vi "Error - Fire Error.vi"(8 "error in (no error)":errorcluster, 10 "Error Type":T1, 11 "View Model":T2) -> (0 "error out":errorcluster, 3 "View Model":T2)   [LabVIEW 2013]
doc: "Used to send errors to the error handling process."
uses:
  View Model/Controls/View Model.ctl
  Controls/Error Model.ctl
  Controls/Error Types.ctl
  View Model/Controls/Shared Model.ctl
  Elevator Controller/Controls/Elevator Model.ctl
  Elevator Controller/Controls/Controller Overhead.ctl
  Elevator Controller/Controls/Elevator States.ctl
  Elevator Controller/Controls/Elevator Location.ctl
  Elevator Controller/Controls/Elevator Command Event.ctl
  Elevator Controller/Controls/Elevator Commands.ctl
  Configuration/Controls/Configuration Model.ctl
  Configuration/Controls/Configuration Data.ctl
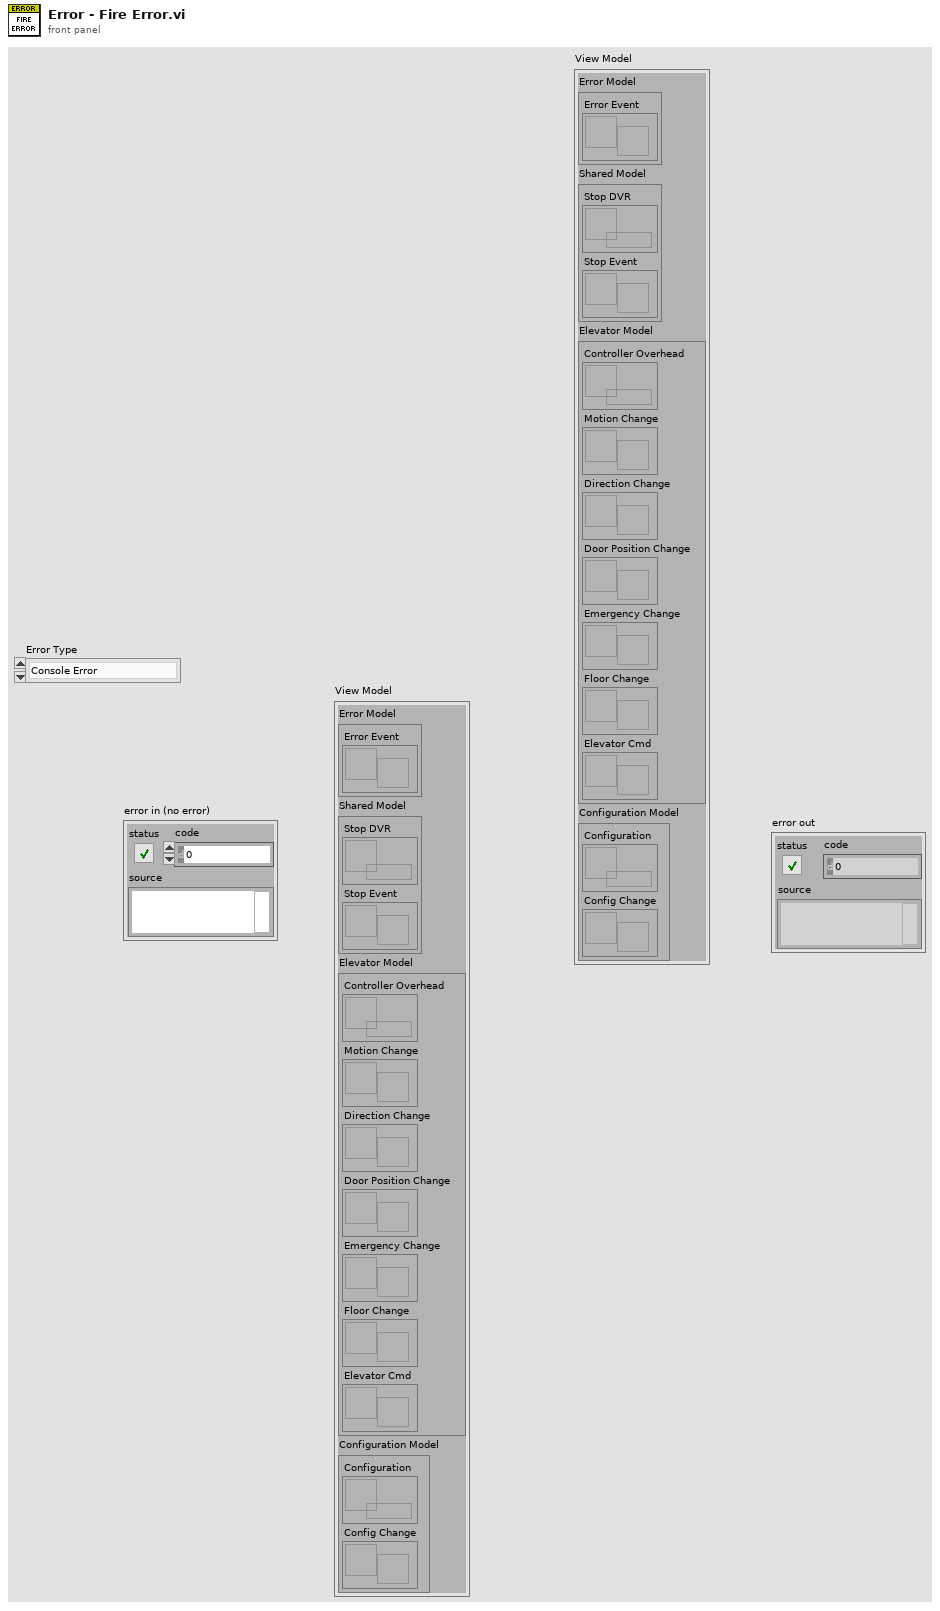
[diagram p1: front panel]
types:
  T1 = typedef "Error Types.ctl" = enum16{"Console Error", "Process Step Error", "Sensor Interface IO Error"}
  T2 = typedef "View Model.ctl" = cluster{"Error Model":T3, "Shared Model":T4, "Elevator Model":T5, "Configuration Model":T6}
  T3 = typedef "Error Model.ctl" = cluster{"Error Event":refnum<user-event>}
  T4 = typedef "Shared Model.ctl" = cluster{"Stop DVR":refnum<data-value>, "Stop Event":refnum<user-event>}
  T5 = typedef "Elevator Model.ctl" = cluster{"Controller Overhead":refnum<data-value>, "Motion Change":refnum<user-event>, "Direction Change":refnum<user-event>, "Door Position Change":refnum<user-event>, "Emergency Change":refnum<user-event>, "Floor Change":refnum<user-event>, "Elevator Cmd":refnum<user-event>}
  T6 = typedef "Configuration Model.ctl" = cluster{"Configuration":refnum<data-value>, "Config Change":refnum<user-event>}
  T7 = cluster{"Error Type":T1, "error in (no error)":errorcluster}
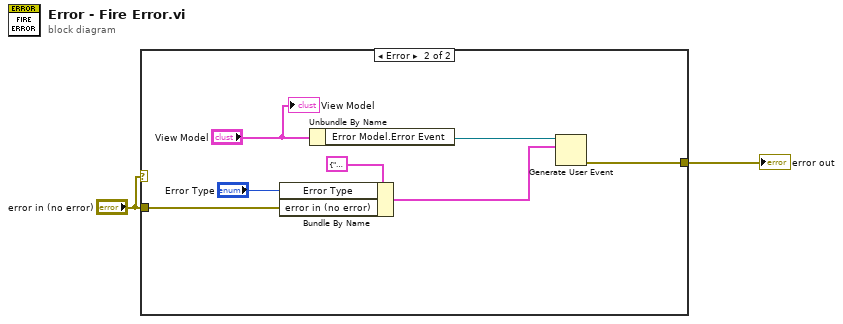
[diagram p0: block diagram]
diagram:
  n1 = case shown="Error" "error in (no error)" {
    tunnel: "error in (no error)" -> [w3 w7]
    tunnel: [w3 w5] -> w2
    frame No Error {
    }
    frame Error {
      n2 = Bundle By Name(cluster=T7 {"Error Type"=enum."Console Error", "error in (no error)"={"status"=FALSE, "code"=0, "source"=""}} ("event data"), "Error Type"="Error Type", "error in (no error)"=w7) -> (w6:T7)
      n3 = Unbundle By Name("View Model") -> ("Error Model.Error Event"=w10:refnum<user-event>)
      n4 = Generate User Event(user event=w10, event data cluster=w6) -> (error out=w5:errorcluster)  [unwired: 2 in, 1 out]
      "View Model" <- "View Model"
    }
  }
  "error out" <- w2
